vi "Get_LabVIEW_printing_method_setting.vi"(0 "error in (no error)":errorcluster) -> (1 "Print method":T1 items=["Unchanged", "Standard", "PostScript", "Bitmap"], 2 "error out":errorcluster)   [LabVIEW 2020, in "NI_ReportGenerationCore.lvlib"]
uses:
  <vilib>/Utility/NIReport.llb/NI_ReportGenerationCore.lvlib
  <vilib>/printing/EasyPrintingControls.llb/printing_method.ctl
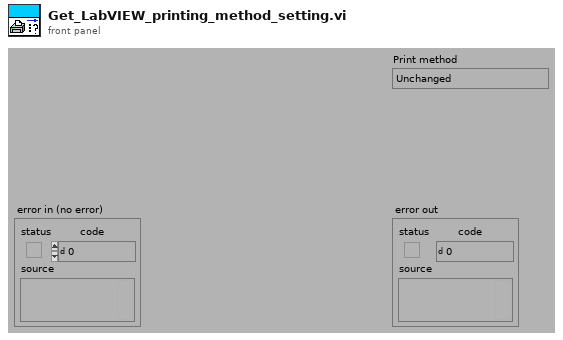
[diagram p1: front panel]
types:
  T1 = typedef "NI_ReportGenerationCore.lvlib/printing_method.ctl" = u16
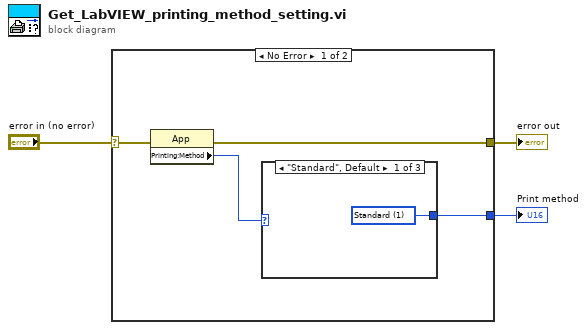
[diagram p0: block diagram]
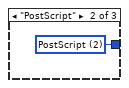
[diagram p2: hidden frame]
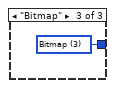
[diagram p3: hidden frame]
diagram:
  n1 = case shown="No Error" "error in (no error)" {
    selector: "error in (no error)" -> [w6 w11]
    tunnel: [w7 w11] -> w3
    tunnel: [w4 _] -> w1
    frame No Error {
      n2 = property class="App"(error in=w6) -> (error out=w7:errorcluster, "Printing:Method"=w5:enum32{"Standard", "PostScript", "Bitmap"})  [unwired: 1 in, 1 out]
      n3 = case shown="\"Standard\", Default" w5 {
        tunnel: [w8 w9 w10] -> w4
        frame "Standard", Default {
          w8 = T1 1 items=["Unchanged", "Standard", "PostScript", "Bitmap"] ("printing method")
        }
        frame "PostScript" {
          w9 = T1 2 items=["Unchanged", "Standard", "PostScript", "Bitmap"] ("printing method")
        }
        frame "Bitmap" {
          w10 = T1 3 items=["Unchanged", "Standard", "PostScript", "Bitmap"] ("printing method")
        }
      }
    }
    frame Error {
    }
  }
  "error out" <- w3
  "Print method" <- w1
